vi "WLAN - niVST - RFSG - Generate Script.vi"(0 "Initial Delay (ms)":dbl, 5 "Number of Packets":i32=50 min=1 max=1000, 7 "Number of Scripts":i32) -> (4 "Array":string[](array[string]))   [LabVIEW 2011]
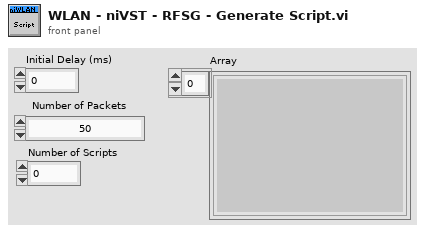
[diagram p1: front panel]
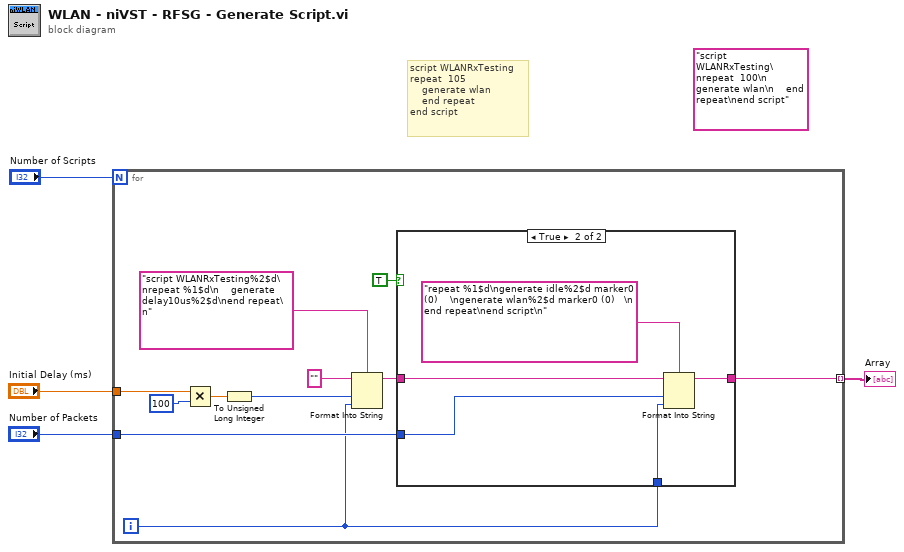
[diagram p0: block diagram]
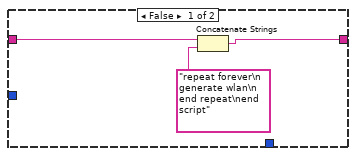
[diagram p2: hidden frame]
diagram:
  (unwired) "script WLANRxTesting\nrepeat  100\n    generate wlan\n    end repeat\nend script" ("Script")
  # "script WLANRxTesting\nrepeat  105\n    generate wlan\n    end repeat\nend script"
  n1 = for {
    N: "Number of Scripts" -> [_]
    tunnel: "Number of Packets" -> [w13]
    tunnel: "Initial Delay (ms)" -> [w12]
    tunnel: [w8] -> w1 mode=indexing
    i -> [w9]
    n2 = Multiply(x=w12, y=u32 100) -> (x*y=w7:dbl)
    n3 = To Unsigned Long Integer(number=w7) -> (unsigned 32bit integer=w6:u32)
    n4 = Format Into String(format string="script WLANRxTesting%2$d\nrepeat %1$d\n    generate delay10us%2$d\nend repeat\n" ("Script"), initial string="", w6, w9) -> (resulting string=w14:string)  [unwired: 1 in, 1 out]
    n5 = case shown="True" TRUE {
      tunnel: w14 -> [w18 w23]
      tunnel: w13 -> [_ w22]
      tunnel: [w16 w20] -> w8
      tunnel: w9 -> [_ w19]
      frame False {
        n6 = Concatenate Strings(w18, "repeat forever\n    generate wlan\n    end repeat\nend script" ("Script")) -> (w16:string)
      }
      frame True {
        n7 = Format Into String(format string="repeat %1$d\ngenerate idle%2$d marker0 (0)    \ngenerate wlan%2$d marker0 (0)   \n    end repeat\nend script\n" ("Script"), initial string=w23, w22, w19) -> (resulting string=w20:string)  [unwired: 1 in, 1 out]
      }
    }
  }
  "Array" <- w1
